vi "Read Serial Data.vi"(0 "FPGA Main IN":refnum<k20>, 5 "Serial Data IN":T1, 11 "Error IN":errorcluster) -> (4 "FPGA VI OUT":refnum<k20>, 6 "Serial Data Out":T1, 15 "Error OUT":errorcluster)   [LabVIEW 2011]
uses:
  Host/Driver/Serial RS485/Controls/Serial Data Cluster.ctl
  <vilib>/Utility/error.llb/Error Cluster From Error Code.vi
  <vilib>/rvi/errors/niLvFpgaAdjustHostInterfaceError.vi
  <vilib>/RVI Host/nirviSupport.llb/nirviErrorClusterFromErrorCode.vi
  <vilib>/rvi/interface/nirviReadWriteControl/nirviReadWriteControl.xnode
  FPGA Bitfiles/JAGM_FPGATarget_FPGAMain_A31A659D.lvbitx
  FPGA Source/FPGA Main.vi
  <vilib>/rvi/interface/nirviMethod/nirviMethod.xnode
  NiFpgaLv.dll
  <vilib>/rvi/interface/nirviMethod/StockFPGA_InlinedMethodWaitForSingleIRQ.vi
  <vilib>/FPGAPlugInAG/sbRIO-9606/niLvFpga_WaitOnIrq_sbRIO-9606.vi
  <vilib>/FPGAPlugInAG/sbRIO-9606/niLvFpga_ReadFifo_sbRIO-9606.vi
  <vilib>/rvi/errors/niLvFpgaMergeErrorWithErrorCode.vi
  <vilib>/FPGAPlugInAG/sbRIO-9606/niLvFpga_AcknowledgeIrq_sbRIO-9606.vi
panel:
  out "String_Chan_4":string
  out "#of Element Read Chan _4":i32
  out "String_Chan_3":string
  out "#of Element Read Chan _3":i32
  out "String_Chan_2":string
  out "#of Element Read Chan _2":i32
  out "#of Element Read Chan _1":i32
  out "String_Chan_1":string
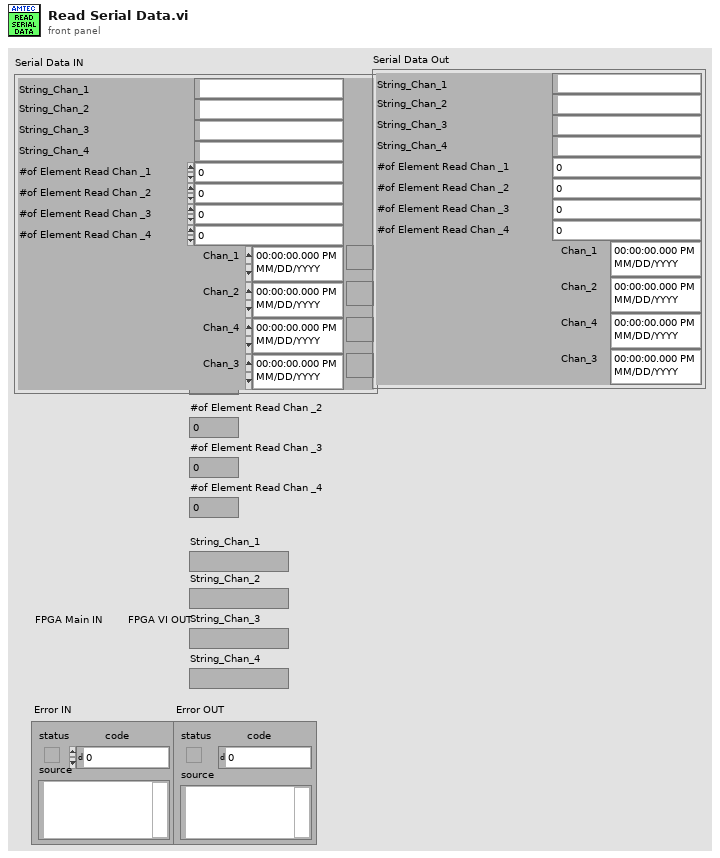
[diagram p1: front panel]
types:
  T1 = typedef "Serial Data Cluster.ctl" = cluster{"String_Chan_1":string, "String_Chan_2":string, "String_Chan_3":string, "String_Chan_4":string, "#of Element Read Chan _1":i32, "#of Element Read Chan _2":i32, "#of Element Read Chan _3":i32, "#of Element Read Chan _4":i32, "Chan_1":timestamp, "Chan_2":timestamp, "Chan_3":timestamp, "Chan_4":timestamp}
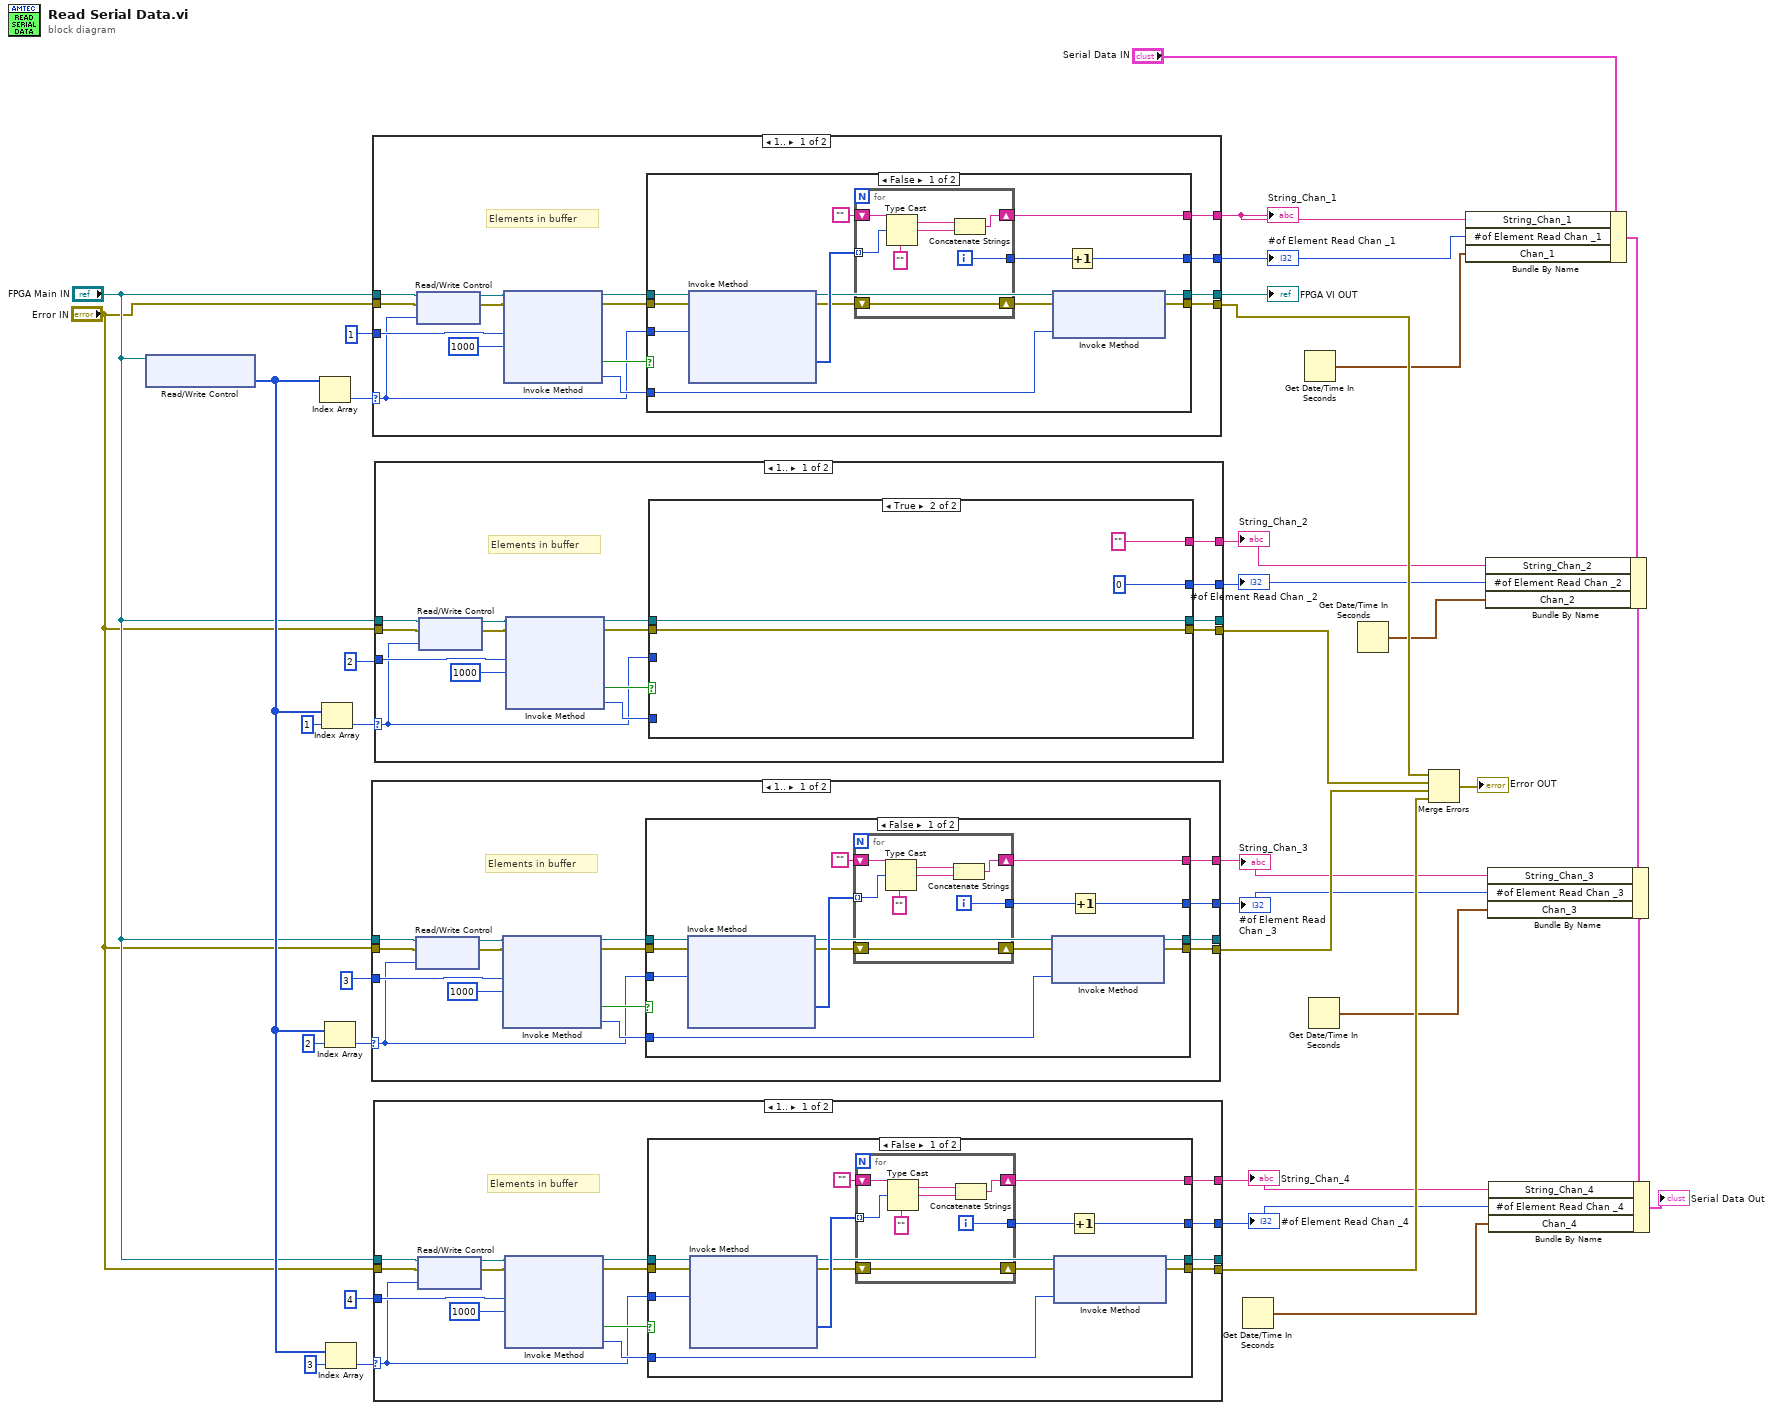
[diagram p0: block diagram]
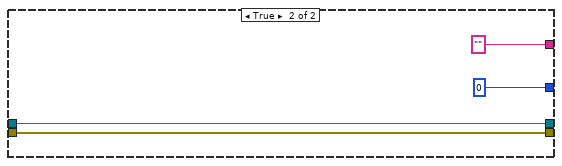
[diagram p2: hidden frame]
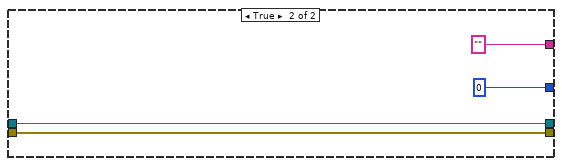
[diagram p4: hidden frame]
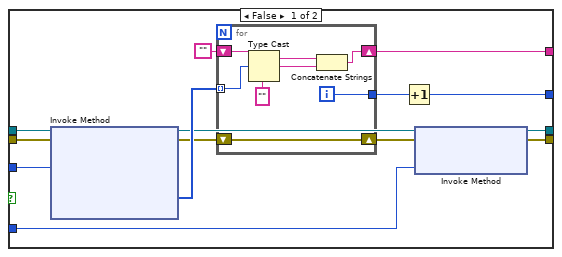
[diagram p6: hidden frame]
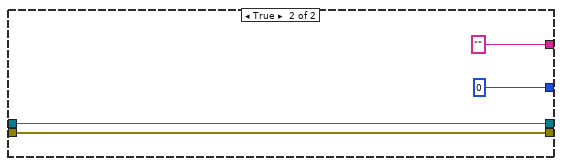
[diagram p8: hidden frame]
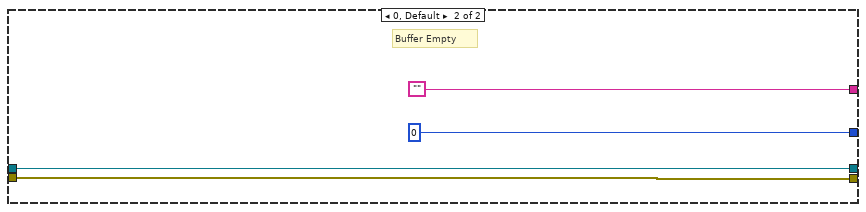
[diagram p9: hidden frame]
diagram:
  n1 = xnode "Read/Write Control"("FPGA VI Reference In"="FPGA Main IN") -> ("Element in Buffer"=w30:u32[])  [unwired: 1 in, 2 out]
  n2 = Index Array(array=w30) -> (element=w35:u32)  [unwired: 1 in]
  n3 = Index Array(array=w30, index=1) -> (element=w34:u32)
  n4 = Index Array(array=w30, index=2) -> (element=w18:u32)
  n5 = Index Array(array=w30, index=3) -> (element=w19:u32)
  n6 = case shown="1.." w18 {
    selector: w18 -> [w38 _]
    tunnel: "FPGA Main IN" -> [w42 w81]
    tunnel: "Error IN" -> [w41 w80]
    tunnel: [w50 w81] -> _
    tunnel: [w51 w80] -> w22
    tunnel: [w52 ""] -> w10
    tunnel: 3 ("IRQ Number(s)") -> [w49 _]
    tunnel: [w45 0] -> w9
    frame 1.. {
      # "Elements in buffer"
      n7 = xnode "Read/Write Control"("FPGA VI Reference In"=w42, "error in"=w41, "Buffer#3"=w38) -> ("FPGA VI Reference Out"=w40:refnum<k20>, "error out"=w39:errorcluster)
      n8 = xnode ("Invoke Method")("FPGA VI Reference In"=w40, "error in"=w39, "IRQ Number(s)"=w49, "Timeout (ms)"=1000) -> ("FPGA VI Reference Out"=w47:refnum<k20>, "error out"=w46:errorcluster, "Timed Out"=w44:bool, "IRQ(s) Asserted"=w43:i32)
      n9 = case shown="False" w44 {
        tunnel: [w65 ""] -> w52
        tunnel: w38 -> [w64 _]
        tunnel: [w55 w76] -> w51
        tunnel: [w57 w77] -> w50
        tunnel: w47 -> [w63 w77]
        tunnel: w46 -> [w62 w76]
        tunnel: [w53 0] -> w45
        tunnel: w43 -> [w54 _]
        frame False {
          n10 = xnode ("Invoke Method")("FPGA VI Reference In"=w63, "error in"=w62, "Number of Elements"=w64) -> ("FPGA VI Reference Out"=w58:refnum<k20>, "error out"=w59:errorcluster, "Data"=w61:u8[])  [unwired: 1 in, 1 out]
          n11 = for {
            shift-right: [w73] -> w65
            shift-left: "" -> [w72]
            tunnel: w61 -> [w69] mode=indexing
            tunnel: [w68] -> w60
            shift-right: [w67] -> w56
            shift-left: w59 -> [w67]
            i -> [w68]
            n12 = Type Cast(type="", x=w69) -> (*(type *) &x=w70:string)
            n13 = Concatenate Strings(w72, w70) -> (w73:string)
          }
          n14 = xnode ("Invoke Method")("FPGA VI Reference In"=w58, "error in"=w56, "IRQ Number(s)"=w54) -> ("FPGA VI Reference Out"=w57:refnum<k20>, "error out"=w55:errorcluster)
          n15 = Increment(x=w60) -> (x+1=w53:i32)
        }
        frame True {
        }
      }
    }
    frame 0, Default {
      # "Buffer Empty"
    }
  }
  "String_Chan_3" <- w10
  "#of Element Read Chan _3" <- w9
  n16 = case shown="1.." w35 {
    selector: w35 -> [w82 _]
    tunnel: "FPGA Main IN" -> [w86 w125]
    tunnel: "Error IN" -> [w85 w124]
    tunnel: [w94 w125] -> w37
    tunnel: [w95 w124] -> w24
    tunnel: [w96 ""] -> w16
    tunnel: 1 ("IRQ Number(s)") -> [w93 _]
    tunnel: [w89 0] -> w15
    frame 1.. {
      # "Elements in buffer"
      n17 = xnode "Read/Write Control"("FPGA VI Reference In"=w86, "error in"=w85, "Buffer#1"=w82) -> ("FPGA VI Reference Out"=w84:refnum<k20>, "error out"=w83:errorcluster)
      n18 = xnode ("Invoke Method")("FPGA VI Reference In"=w84, "error in"=w83, "IRQ Number(s)"=w93, "Timeout (ms)"=1000) -> ("FPGA VI Reference Out"=w91:refnum<k20>, "error out"=w90:errorcluster, "Timed Out"=w88:bool, "IRQ(s) Asserted"=w87:i32)
      n19 = case shown="False" w88 {
        tunnel: [w109 ""] -> w96
        tunnel: w82 -> [w108 _]
        tunnel: [w99 w120] -> w95
        tunnel: [w101 w121] -> w94
        tunnel: w91 -> [w107 w121]
        tunnel: w90 -> [w106 w120]
        tunnel: [w97 0] -> w89
        tunnel: w87 -> [w98 _]
        frame False {
          n20 = xnode ("Invoke Method")("FPGA VI Reference In"=w107, "error in"=w106, "Number of Elements"=w108) -> ("FPGA VI Reference Out"=w102:refnum<k20>, "error out"=w103:errorcluster, "Data"=w105:u8[])  [unwired: 1 in, 1 out]
          n21 = for {
            shift-right: [w117] -> w109
            shift-left: "" -> [w116]
            tunnel: w105 -> [w113] mode=indexing
            tunnel: [w112] -> w104
            shift-right: [w111] -> w100
            shift-left: w103 -> [w111]
            i -> [w112]
            n22 = Type Cast(type="", x=w113) -> (*(type *) &x=w114:string)
            n23 = Concatenate Strings(w116, w114) -> (w117:string)
          }
          n24 = xnode ("Invoke Method")("FPGA VI Reference In"=w102, "error in"=w100, "IRQ Number(s)"=w98) -> ("FPGA VI Reference Out"=w101:refnum<k20>, "error out"=w99:errorcluster)
          n25 = Increment(x=w104) -> (x+1=w97:i32)
        }
        frame True {
        }
      }
    }
    frame 0, Default {
      # "Buffer Empty"
    }
  }
  "String_Chan_1" <- w16
  "FPGA VI OUT" <- w37
  "#of Element Read Chan _1" <- w15
  n26 = case shown="1.." w19 {
    selector: w19 -> [w126 _]
    tunnel: "FPGA Main IN" -> [w130 w169]
    tunnel: "Error IN" -> [w129 w168]
    tunnel: [w138 w169] -> _
    tunnel: [w139 w168] -> w21
    tunnel: [w140 ""] -> w7
    tunnel: 4 ("IRQ Number(s)") -> [w137 _]
    tunnel: [w133 0] -> w6
    frame 1.. {
      # "Elements in buffer"
      n27 = xnode "Read/Write Control"("FPGA VI Reference In"=w130, "error in"=w129, "Buffer#4"=w126) -> ("FPGA VI Reference Out"=w128:refnum<k20>, "error out"=w127:errorcluster)
      n28 = xnode ("Invoke Method")("FPGA VI Reference In"=w128, "error in"=w127, "IRQ Number(s)"=w137, "Timeout (ms)"=1000) -> ("FPGA VI Reference Out"=w135:refnum<k20>, "error out"=w134:errorcluster, "Timed Out"=w132:bool, "IRQ(s) Asserted"=w131:i32)
      n29 = case shown="False" w132 {
        tunnel: [w153 ""] -> w140
        tunnel: w126 -> [w152 _]
        tunnel: [w143 w164] -> w139
        tunnel: [w145 w165] -> w138
        tunnel: w135 -> [w151 w165]
        tunnel: w134 -> [w150 w164]
        tunnel: [w141 0] -> w133
        tunnel: w131 -> [w142 _]
        frame False {
          n30 = xnode ("Invoke Method")("FPGA VI Reference In"=w151, "error in"=w150, "Number of Elements"=w152) -> ("FPGA VI Reference Out"=w146:refnum<k20>, "error out"=w147:errorcluster, "Data"=w149:u8[])  [unwired: 1 in, 1 out]
          n31 = for {
            shift-right: [w161] -> w153
            shift-left: "" -> [w160]
            tunnel: w149 -> [w157] mode=indexing
            tunnel: [w156] -> w148
            shift-right: [w155] -> w144
            shift-left: w147 -> [w155]
            i -> [w156]
            n32 = Type Cast(type="", x=w157) -> (*(type *) &x=w158:string)
            n33 = Concatenate Strings(w160, w158) -> (w161:string)
          }
          n34 = xnode ("Invoke Method")("FPGA VI Reference In"=w146, "error in"=w144, "IRQ Number(s)"=w142) -> ("FPGA VI Reference Out"=w145:refnum<k20>, "error out"=w143:errorcluster)
          n35 = Increment(x=w148) -> (x+1=w141:i32)
        }
        frame True {
        }
      }
    }
    frame 0, Default {
      # "Buffer Empty"
    }
  }
  "String_Chan_4" <- w7
  "#of Element Read Chan _4" <- w6
  n36 = case shown="1.." w34 {
    selector: w34 -> [w170 _]
    tunnel: "FPGA Main IN" -> [w174 w213]
    tunnel: "Error IN" -> [w173 w212]
    tunnel: [w182 w213] -> _
    tunnel: [w183 w212] -> w23
    tunnel: [w184 ""] -> w13
    tunnel: 2 ("IRQ Number(s)") -> [w181 _]
    tunnel: [w177 0] -> w12
    frame 1.. {
      # "Elements in buffer"
      n37 = xnode "Read/Write Control"("FPGA VI Reference In"=w174, "error in"=w173, "Buffer#2"=w170) -> ("FPGA VI Reference Out"=w172:refnum<k20>, "error out"=w171:errorcluster)
      n38 = xnode ("Invoke Method")("FPGA VI Reference In"=w172, "error in"=w171, "IRQ Number(s)"=w181, "Timeout (ms)"=1000) -> ("FPGA VI Reference Out"=w179:refnum<k20>, "error out"=w178:errorcluster, "Timed Out"=w176:bool, "IRQ(s) Asserted"=w175:i32)
      n39 = case shown="True" w176 {
        tunnel: [w197 ""] -> w184
        tunnel: w170 -> [w196 _]
        tunnel: [w187 w208] -> w183
        tunnel: [w189 w209] -> w182
        tunnel: w179 -> [w195 w209]
        tunnel: w178 -> [w194 w208]
        tunnel: [w185 0] -> w177
        tunnel: w175 -> [w186 _]
        frame False {
          n40 = xnode ("Invoke Method")("FPGA VI Reference In"=w195, "error in"=w194, "Number of Elements"=w196) -> ("FPGA VI Reference Out"=w190:refnum<k20>, "error out"=w191:errorcluster, "Data"=w193:u8[])  [unwired: 1 in, 1 out]
          n41 = for {
            shift-right: [w205] -> w197
            shift-left: "" -> [w204]
            tunnel: w193 -> [w201] mode=indexing
            tunnel: [w200] -> w192
            shift-right: [w199] -> w188
            shift-left: w191 -> [w199]
            i -> [w200]
            n42 = Type Cast(type="", x=w201) -> (*(type *) &x=w202:string)
            n43 = Concatenate Strings(w204, w202) -> (w205:string)
          }
          n44 = Increment(x=w192) -> (x+1=w185:i32)
          n45 = xnode ("Invoke Method")("FPGA VI Reference In"=w190, "error in"=w188, "IRQ Number(s)"=w186) -> ("FPGA VI Reference Out"=w189:refnum<k20>, "error out"=w187:errorcluster)
        }
        frame True {
        }
      }
    }
    frame 0, Default {
      # "Buffer Empty"
    }
  }
  "String_Chan_2" <- w13
  "#of Element Read Chan _2" <- w12
  n46 = Get Date/Time In Seconds() -> (seconds since 1Jan1904=w2:timestamp)
  n47 = Get Date/Time In Seconds() -> (seconds since 1Jan1904=w1:timestamp)
  n48 = Get Date/Time In Seconds() -> (seconds since 1Jan1904=w3:timestamp)
  n49 = Get Date/Time In Seconds() -> (seconds since 1Jan1904=w4:timestamp)
  n50 = Merge Errors(w24, w23, w22, w21) -> (→"Error OUT":errorcluster)
  n51 = Bundle By Name(cluster="Serial Data IN", "String_Chan_1"=w16, "#of Element Read Chan _1"=w15, "Chan_1"=w1) -> (w14:T1)
  n52 = Bundle By Name(cluster=w14, "String_Chan_2"=w13, "#of Element Read Chan _2"=w12, "Chan_2"=w4) -> (w11:T1)
  n53 = Bundle By Name(cluster=w11, "String_Chan_3"=w10, "#of Element Read Chan _3"=w9, "Chan_3"=w3) -> (w8:T1)
  n54 = Bundle By Name(cluster=w8, "String_Chan_4"=w7, "#of Element Read Chan _4"=w6, "Chan_4"=w2) -> (→"Serial Data Out":T1)
